vi "Dispense FN - ON - Setpoints - Dynamic (SubVI).vi"(0 "Settings":T1={"ON Settings"={"Enable Dynamic Setpoint?"=TRUE, "Enable Dynamic Dispense Time?"=TRUE, "Enable Drain Rate Functions"=TRUE, "Dispense Sample Time (s)"=0.5, "Dispense Slope Ave"=0, "ON Timeout (sec)"=600.0, "1st Setpoint (% of Target)"=0.0, "2nd Setpoint (% of Target)"=0.0, "3rd Setpoint (% of Target)"=0.0, "Measure Dispense Delay (sec)"=0.0, "Settle Slope Sample Time (s)"=0.0}, "OFF Settings"={"Drain Sample Time (s)"=0.5, "Drain Rate Ave Size"=5, "Drain Rate Limits (± g/sec)"=10.0, "Level Slope Range (± g/sec)"=0.25, "OFF Timeout (sec)"=0.0, "Near SP Slope Level (± g/sec)"=0.01, "Near Setpoint Threshold (%)"=95.0}, "Overshoot Settings"={"Time Limit (s)"=60.0, "Container MAX (g)"=1500.0, "Max FILL Slope (+/- g/sec)"=10.0, "% Overshot to Enable (>)"=0.25}, "FILL Timeout (s)"=300.0, "Full Settle Time (s)"=3.0, "Pre-Hydrate \nSpray Time (s)"=10.0, "Pre-Hydrate \nWait Time (s)"=30.0}, 2 "Measured Mass (g)":dbl, 4 "State Change?":bool, 5 "Main Case Change?":bool, 7 "Drain Mass Gain (g)":dbl, 9 "Static Setpoint (g)":dbl, 11 "Spray Mass Loss (g)":dbl) -> (14 "Spray Count":i32, 16 "Dynamic Setpoint (g)":dbl)   [LabVIEW 2009]
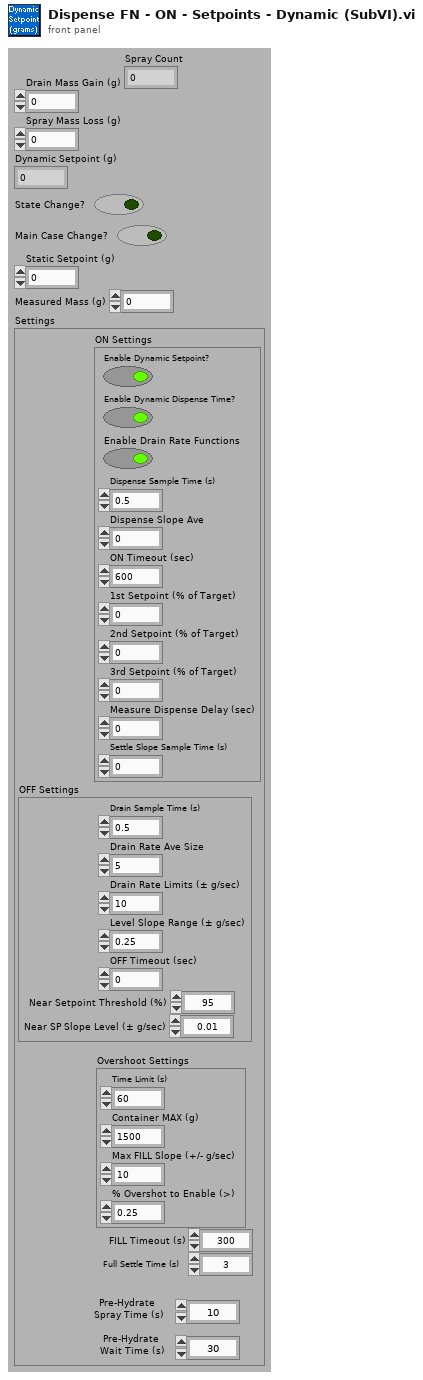
[diagram p1: front panel]
types:
  T1 = cluster{"ON Settings":cluster{"Enable Dynamic Setpoint?":bool, "Enable Dynamic Dispense Time?":bool, "Enable Drain Rate Functions":bool, "Dispense Sample Time (s)":dbl, "Dispense Slope Ave":i32, "ON Timeout (sec)":dbl, "1st Setpoint (% of Target)":dbl, "2nd Setpoint (% of Target)":dbl, "3rd Setpoint (% of Target)":dbl, "Measure Dispense Delay (sec)":dbl, "Settle Slope Sample Time (s)":dbl}, "OFF Settings":cluster{"Drain Sample Time (s)":dbl, "Drain Rate Ave Size":i32, "Drain Rate Limits (± g/sec)":dbl, "Level Slope Range (± g/sec)":dbl, "OFF Timeout (sec)":dbl, "Near SP Slope Level (± g/sec)":dbl, "Near Setpoint Threshold (%)":dbl}, "Overshoot Settings":cluster{"Time Limit (s)":dbl, "Container MAX (g)":dbl, "Max FILL Slope (+/- g/sec)":dbl, "% Overshot to Enable (>)":dbl}, "FILL Timeout (s)":dbl, "Full Settle Time (s)":dbl, "Pre-Hydrate \nSpray Time (s)":dbl, "Pre-Hydrate \nWait Time (s)":dbl}
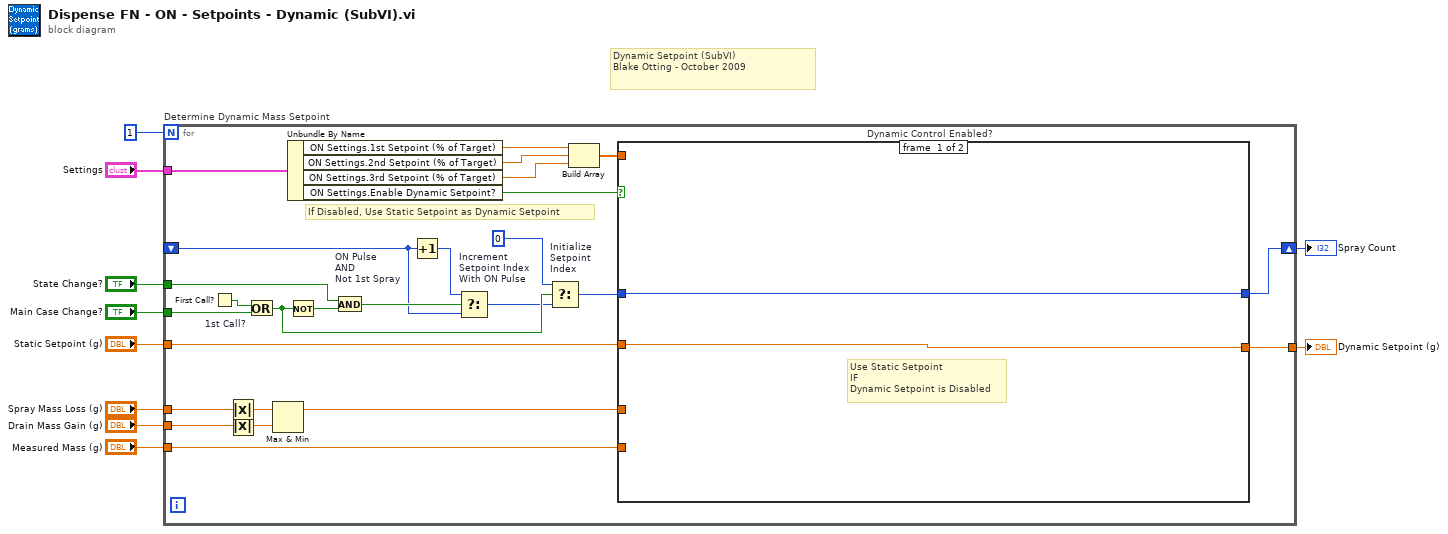
[diagram p0: block diagram]
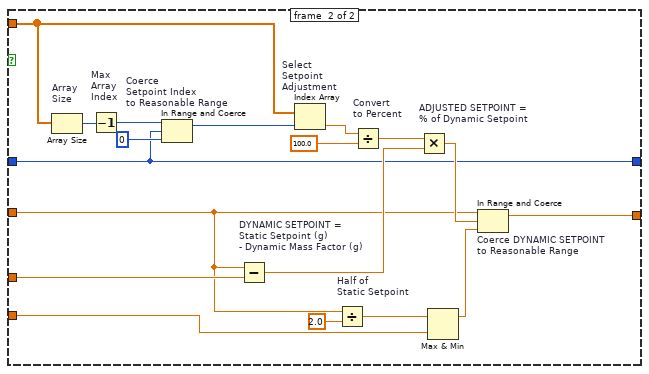
[diagram p2: hidden frame]
diagram:
  # "Dynamic Setpoint (SubVI)\nBlake Otting - October 2009"
  n1 = for "Determine Dynamic Mass Setpoint" {
    N: 1 -> [_]
    tunnel: "Measured Mass (g)" -> [w11]
    tunnel: "Main Case Change?" -> [w30]
    shift-right: [w35] -> w1
    shift-left: _ -> [w24]
    tunnel: "State Change?" -> [w12]
    tunnel: "Static Setpoint (g)" -> [w28]
    tunnel: [w27] -> w9
    tunnel: "Spray Mass Loss (g)" -> [w23]
    tunnel: "Drain Mass Gain (g)" -> [w22]
    tunnel: "Settings" -> [w17]
    # "If Disabled, Use Static Setpoint as Dynamic Setpoint"
    n2 = First Call? "1st Call?"() -> (First Call?: T/F=w29:bool)
    n3 = Absolute Value(x=w23) -> (abs(x)=w14:dbl)
    n4 = Absolute Value(x=w22) -> (abs(x)=w13:dbl)
    n5 = Or(x=w29, y=w30) -> (x .or. y?=w31:bool)
    n6 = Max & Min(x=w14, y=w13) -> (max(x,y)=w21:dbl)  [unwired: 1 out]
    n7 = Unbundle By Name(w17) -> ("ON Settings.1st Setpoint (% of Target)"=w18:dbl, "ON Settings.2nd Setpoint (% of Target)"=w19:dbl, "ON Settings.3rd Setpoint (% of Target)"=w20:dbl, "ON Settings.Enable Dynamic Setpoint?"=w15:bool)
    n8 = Not(x=w31) -> (.not. x?=w32:bool)
    n9 = And "ON Pulse\nAND\nNot 1st Spray"(x=w12, y=w32) -> (x .and. y?=w33:bool)
    n10 = Increment(x=w24) -> (x+1=w34:i32)
    n11 = Select "Increment\nSetpoint Index\nWith ON Pulse"(t=w34, s=w33, f=w24) -> (s? t:f=w25:i32)
    n12 = Select "Initialize\nSetpoint\nIndex"(t=0, s=w31, f=w25) -> (s? t:f=w26:i32)
    n13 = Build Array(w18, w19, w20) -> (w16:dbl[])
    n14 = case "Dynamic Control Enabled?" shown="True" w15 {
      tunnel: w28 -> [w37 w43]
      tunnel: [w37 w55] -> w27
      tunnel: w26 -> [w38 w44]
      tunnel: [w38 w44] -> w35
      tunnel: w16 -> [_ w49]
      tunnel: w11 -> [_ w41]
      tunnel: w21 -> [_ w53]
      frame #0 {
        # "Use Static Setpoint\nIF \nDynamic Setpoint is Disabled"
      }
      frame #1 {
        n15 = Array Size "Array\nSize"(array=w49) -> (size(s)=w48:i32)
        n16 = Decrement "Max\nArray\nIndex"(x=w48) -> (x-1=w47:i32)
        n17 = In Range and Coerce "Coerce \nSetpoint Index\nto Reasonable Range"(upper limit=w47, x=w44, lower limit=0) -> (coerced(x)=w45:i32)  [unwired: 1 out]
        n18 = Subtract "DYNAMIC SETPOINT =\nStatic Setpoint (g)\n- Dynamic Mass Factor (g)"(x=w43, y=w53) -> (x-y=w52:dbl)
        n19 = Index Array "Select\nSetpoint\nAdjustment"(array=w49, index=w45) -> (element=w56:dbl)
        n20 = Divide "Half of\nStatic Setpoint"(x=w43, y=2.0) -> (x/y=w40:dbl)
        n21 = Divide "Convert\nto Percent"(x=w56, y=100.0) -> (x/y=w51:dbl)
        n22 = Multiply "ADJUSTED SETPOINT = \n% of Dynamic Setpoint"(x=w51, y=w52) -> (x*y=w50:dbl)
        n23 = Max & Min(x=w40, y=w41) -> (max(x,y)=w39:dbl)  [unwired: 1 out]
        n24 = In Range and Coerce "Coerce DYNAMIC SETPOINT\nto Reasonable Range"(upper limit=w43, x=w50, lower limit=w39) -> (coerced(x)=w55:dbl)  [unwired: 1 out]
      }
    }
  }
  "Dynamic Setpoint (g)" <- w9
  "Spray Count" <- w1
